vi "op_num_v5.vi"() -> ()   [LabVIEW 2009]
panel:
  out "Putere -W":dbl
  out "Watt-meter":dbl(knob) scale=0.0..12500.0
  in  "Curent":dbl(knob) scale=0.0..50.0
  in  "Tensiune":dbl(knob) scale=0.0..250.0
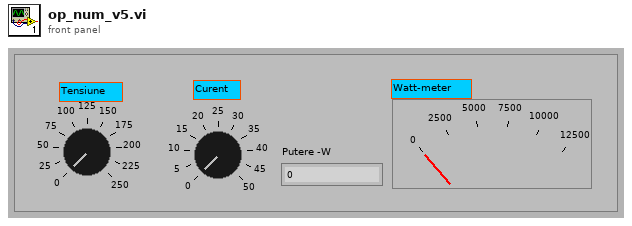
[diagram p1: front panel]
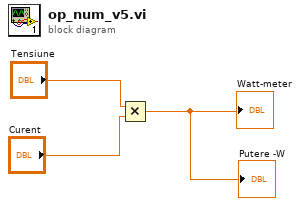
[diagram p0: block diagram]
diagram:
  n1 = Multiply(x="Tensiune", y="Curent") -> (x*y=→"Watt-meter" →"Putere -W":dbl)
